vi "Save Settings to XML.vi"(8 "error in (no error)":errorcluster, 11 "Settings":T1) -> (0 "error out":errorcluster)   [LabVIEW 2018, in "gos Settings.lvlib"]
doc: "Saves the \"User Specified\" configuration data to an XML file. This is used to remember the users settings between executions."
uses:
  gos Settings.lvlib
  Settings.ctl
  Acquisition/Hardware Configuration.ctl
  Acquisition/Signal Type.ctl
  Logging/Logging Configuration.ctl
  <vilib>/Utility/xml.llb/Write to XML File(string).vi
  Acquisition/gos Acquisition.lvlib
  Logging/gos Logging.lvlib
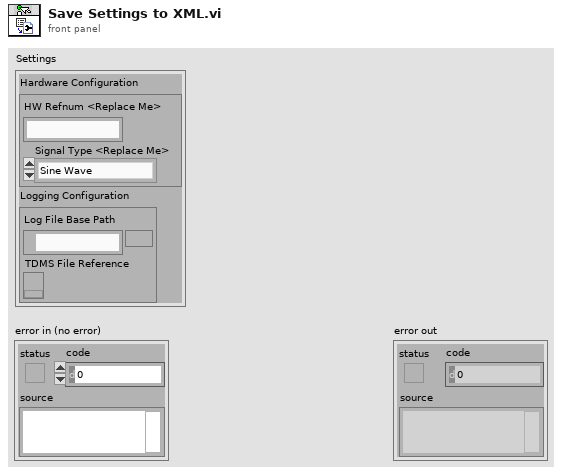
[diagram p1: front panel]
types:
  T1 = typedef "gos Settings.lvlib/Settings.ctl" = cluster{"Hardware Configuration":T2, "Logging Configuration":T4}
  T2 = typedef "gos Acquisition.lvlib/Hardware Configuration.ctl" = cluster{"HW Refnum <Replace Me>":string, "Signal Type <Replace Me>":T3}
  T3 = typedef "gos Acquisition.lvlib/Signal Type.ctl" = enum16{"Sine Wave", "Square with Noise"}
  T4 = typedef "gos Logging.lvlib/Logging Configuration.ctl" = cluster{"Log File Base Path":path, "TDMS File Reference":refnum<k34>}
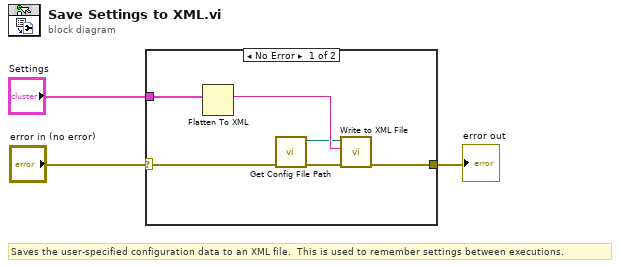
[diagram p0: block diagram]
diagram:
  # "Saves the user-specified configuration data to an XML file.  This is used to remember settings between executions."
  n1 = case shown="No Error" "error in (no error)" {
    selector: "error in (no error)" -> [w5 w10]
    tunnel: [w7 w10] -> w2
    tunnel: "Settings" -> [w9 _]
    frame No Error {
      n2 = Flatten To XML(anything=w9) -> (xml string=w8:string)
      n3 = call "Get Config File Path.vi"("error in (no error)"=w5) -> ("error out"=w4:errorcluster, "XML File Path"=w6:path)  [unwired: 9 in]
      n4 = call-poly <vilib>:"Write to XML File.vi"("error in (no error)"=w4, "XML Input"=w8, "XML File Path"=w6) -> ("error out"=w7:errorcluster)  [unwired: 6 in, 2 out]
    }
    frame Error {
    }
  }
  "error out" <- w2
